vi "toml_api_remove_section.vi"(7 "resolved path":path, 8 "error in (no error)":errorcluster, 10 "section":string, 11 "vi in":refnum<vi>) -> (0 "error out":errorcluster, 2 "section exists":bool, 3 "vi out":refnum<vi>)   [LabVIEW 2017]
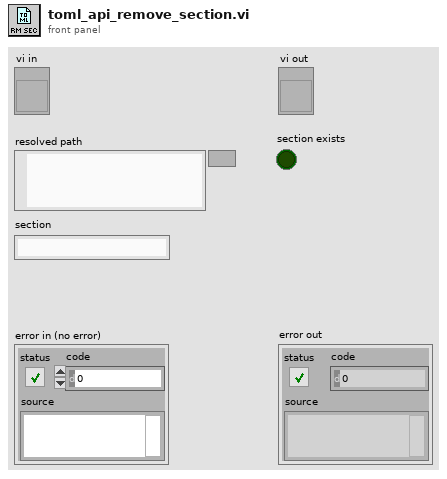
[diagram p1: front panel]
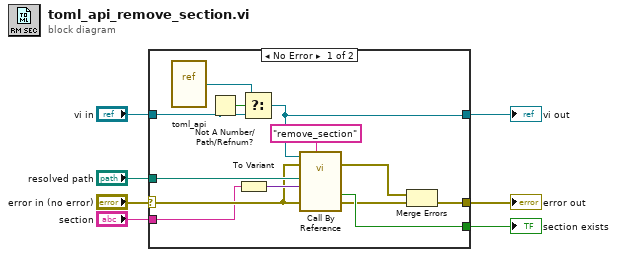
[diagram p0: block diagram]
diagram:
  n1 = case shown="No Error" "error in (no error)" {
    selector: "error in (no error)" -> [w11 w22]
    tunnel: [w19 _] -> w7
    tunnel: "resolved path" -> [w17 _]
    tunnel: [w13 w22] -> w5
    tunnel: "vi in" -> [w10 w21]
    tunnel: [w9 w21] -> w2
    tunnel: "section" -> [w8 _]
    frame No Error {
      n2 = vi-ref "toml_api.vi"() -> (w16:refnum<vi>)
      n3 = Not A Number/Path/Refnum?(number/path/refnum=w10) -> (NaN/Path/Refnum?=w15:bool)
      n4 = To Variant(anything=w8) -> (Variant=w20:variant)
      n5 = Select(t=w16, s=w15, f=w10) -> (s? t:f=w9:refnum<vi>)
      n6 = call-by-ref "?"(reference=w9, error in=w11, "cmd"="remove_section", 8:"error in (no error)"=w11, "data in"=w20, "path in"=w17) -> (error out=w12:errorcluster, 0:"error out"=w18:errorcluster, "return"=w19:bool)  [unwired: 4 in, 3 out]
      n7 = Merge Errors(w12, w18) -> (w13:errorcluster)
    }
    frame Error {
    }
  }
  "section exists" <- w7
  "error out" <- w5
  "vi out" <- w2
